vi "Dhoot Front Measurement Block.vi"(0 "Image in":T4, 1 "Coord Centre X":dbl, 2 "Measurement ROI":T10={"Left"=40.0, "Top"=75.0, "Right"=80.0, "Bottom"=3.0, "Angle"=0.0}, 3 "Coord Centre Y":dbl, 4 "Angle":dbl, 5 "ROI Enable":bool, 6 "Measu Ref Step Size":u32=1, 7 "error in (no error)":errorcluster, 8 "Measurement ROI Scan Direction":u16(ring) items=["Left To Right", "Right To Left", "Top To Bottom", "Bottom To Top"], 9 "Measurement Reference ROI":T10={"Left"=0.0, "Top"=0.0, "Right"=0.0, "Bottom"=280.0, "Angle"=0.0}, 10 "Measu ROI Process":T7(ring)=enum."Get First + Last Edge", 11 "Measu Ref Process":T7(ring), 12 "Measu ROI Step Size":u32=1, 13 "Measu Ref Edge Options":T5={"Edge Polarity"=0, "Kernel Size"=5, "Width"=5, "Minimum Edge Strength"=40.0, "Interpolation Type"=enum."Zero Order", "Data Processing Method"=enum."Average"} {"Edge Polarity" items=["All Edges", "Rising Edges", "Falling Edges"]; "Minimum Edge Strength" format="%.2f"; "Width" step=2; "Kernel Size" step=2}, 14 "Measu Edge Options":T5={"Edge Polarity"=0, "Kernel Size"=5, "Width"=5, "Minimum Edge Strength"=40.0, "Interpolation Type"=enum."Zero Order", "Data Processing Method"=enum."Average"} {"Edge Polarity" items=["All Edges", "Rising Edges", "Falling Edges"]; "Minimum Edge Strength" format="%.2f"; "Width" step=2; "Kernel Size" step=2}, 15 "Measu Ref Scan Direction":u16(ring)=2 items=["Left To Right", "Right To Left", "Top To Bottom", "Bottom To Top"], 16 "Calibration Image":T4) -> (18 "Overlay Arrows Lines":T1, 20 "Image out":T4, 21 "Measurement":sgl, 22 "Measu Ref Edge Point":cluster{"X":sgl, "Y":sgl}, 23 "First Edges":T9[](array[typedef]) {"Distance (Real-World)" format="%.2f"; "Location (Real-World)"."Y" format="%.2g"; "Location (Real-World)"."X" format="%.2f"; "Noise" format="%.2f"; "Location (Pixel)"."Y" format="%.2g"; "Location (Pixel)"."X" format="%.2f"; "Strength" format="%.2f"; "Distance (Pixel)" format="%.2f"}, 24 "Last Edges":T9[](array[typedef]) {"Distance (Real-World)" format="%.2f"; "Location (Real-World)"."Y" format="%.2g"; "Location (Real-World)"."X" format="%.2f"; "Noise" format="%.2f"; "Location (Pixel)"."Y" format="%.2g"; "Location (Pixel)"."X" format="%.2f"; "Strength" format="%.2f"; "Distance (Pixel)" format="%.2f"}, 25 "Search Lines":T8[](array[typedef]) {"Edge Info"."Distance (Real-World)" format="%.2f"; "Edge Info"."Location (Real-World)"."Y" format="%.2g"; "Edge Info"."Location (Real-World)"."X" format="%.2f"; "Edge Info"."Noise" format="%.2f"; "Edge Info"."Location (Pixel)"."Y" format="%.2g"; "Edge Info"."Location (Pixel)"."X" format="%.2f"; "Edge Info"."Strength" format="%.2f"; "Edge Info"."Distance (Pixel)" format="%.2f"}, 27 "error IO":errorcluster)   [LabVIEW 2019, in "Algorithm.lvclass"]
uses:
  FrameworkOverrides/Algorithm.lvclass
  <vilib>/vision/NI_Vision_Development_Module.lvlib
  <vilib>/vision/Image Controls.llb/IMAQ Image.ctl
  <vilib>/vision/Measure.llb/Edge New.ctl
  <vilib>/vision/Measure.llb/Search Line.ctl
  <vilib>/vision/Measure.llb/Edge Polarity.ctl
  <vilib>/vision/Measure.llb/Edge Options.ctl
panel:
  out "Second Overlay Line":T2
  out "First Overlay Line":T3
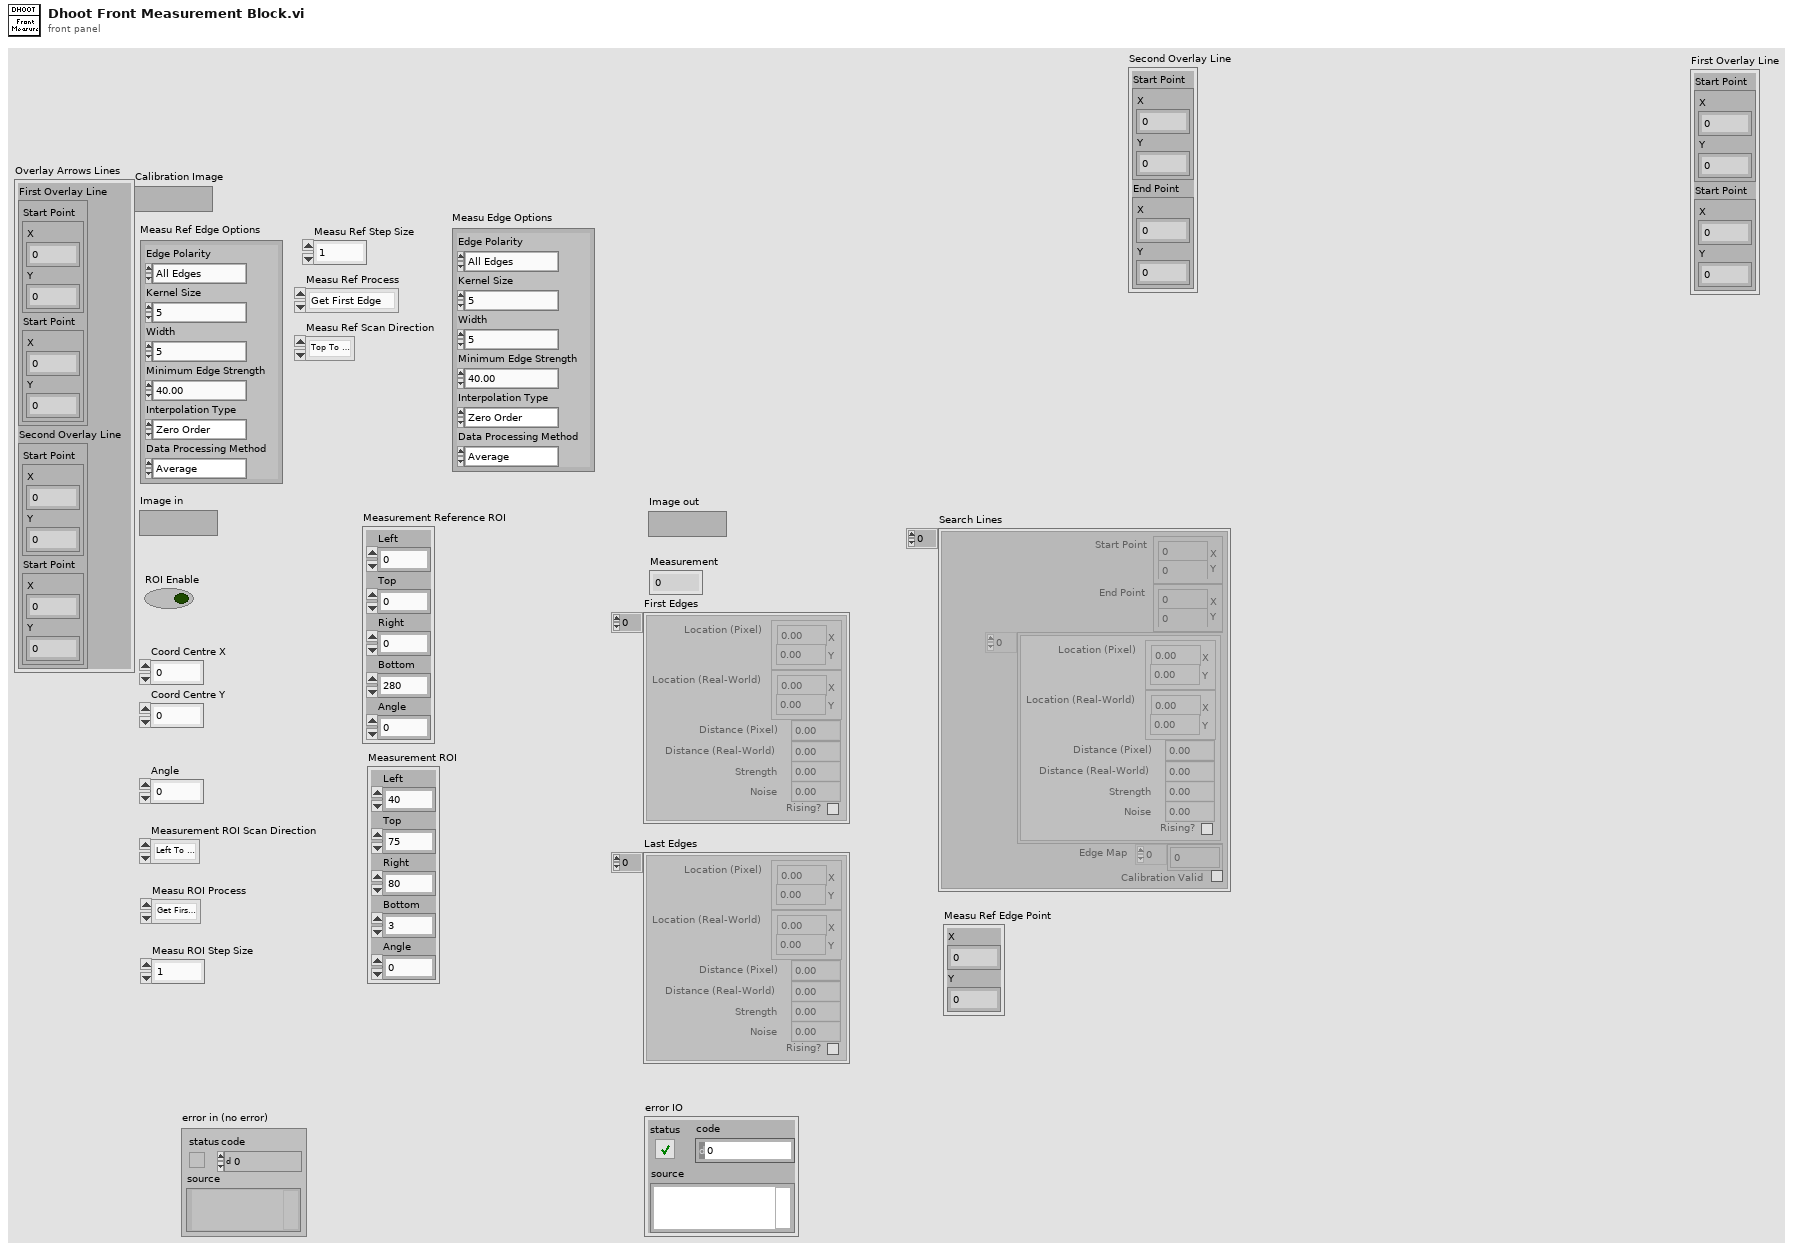
[diagram p1: front panel]
types:
  T1 = cluster{"First Overlay Line ":cluster{"Start Point":cluster{"X":sgl, "Y":sgl}, "Start Point":cluster{"X":sgl, "Y":sgl}}, "Second Overlay Line ":cluster{"Start Point":cluster{"X":sgl, "Y":sgl}, "Start Point":cluster{"X":sgl, "Y":sgl}}}
  T2 = cluster{"Start Point":cluster{"X":sgl, "Y":sgl}, "End Point":cluster{"X":sgl, "Y":sgl}}
  T3 = cluster{"Start Point":cluster{"X":sgl, "Y":sgl}, "Start Point":cluster{"X":sgl, "Y":sgl}}
  T4 = typedef "IMAQ Image.ctl" = refnum<image>
  T5 = typedef "Edge Options.ctl" = cluster{"Edge Polarity":T6, "Kernel Size":u32, "Width":u32, "Minimum Edge Strength":sgl, "Interpolation Type":enum32{"Zero Order", "Bilinear", "Quadratic", "Cubic", "Bilinear Fixed"}, "Data Processing Method":enum32{"Average", "Median"}}
  T6 = typedef "Edge Polarity.ctl" = u32
  T7 = enum16{"Get First Edge", "Get First + Last Edge", "Get All Edges", "Get Best Edge"}
  T8 = typedef "Search Line.ctl" = cluster{"Start Point":cluster{"X":sgl, "Y":sgl}, "End Point":cluster{"X":sgl, "Y":sgl}, "Edge Info":T9[], "Edge Map":dbl[], "Calibration Valid":bool}
  T9 = typedef "Edge New.ctl" = cluster{"Location (Pixel)":cluster{"X":sgl, "Y":sgl}, "Location (Real-World)":cluster{"X":sgl, "Y":sgl}, "Distance (Pixel)":dbl, "Distance (Real-World)":dbl, "Strength":dbl, "Noise":dbl, "Rising?":bool}
  T10 = cluster{"Left":dbl, "Top":dbl, "Right":dbl, "Bottom":dbl, "Angle":dbl}
  T11 = typedef "ROI Descriptor" = cluster{"Global Rectangle":i32[], "Contours":cluster{"ID":enum32{"External", "Internal"}, "Type":u32, "Coordinates":i32[]}[]}
  T12 = cluster{"Start Point":cluster{"X":sgl, "Y":sgl}, "Location (Pixel)":cluster{"X":sgl, "Y":sgl}}
  T13 = cluster{"Location (Pixel)":cluster{"X":sgl, "Y":sgl}, "End Point":cluster{"X":sgl, "Y":sgl}}
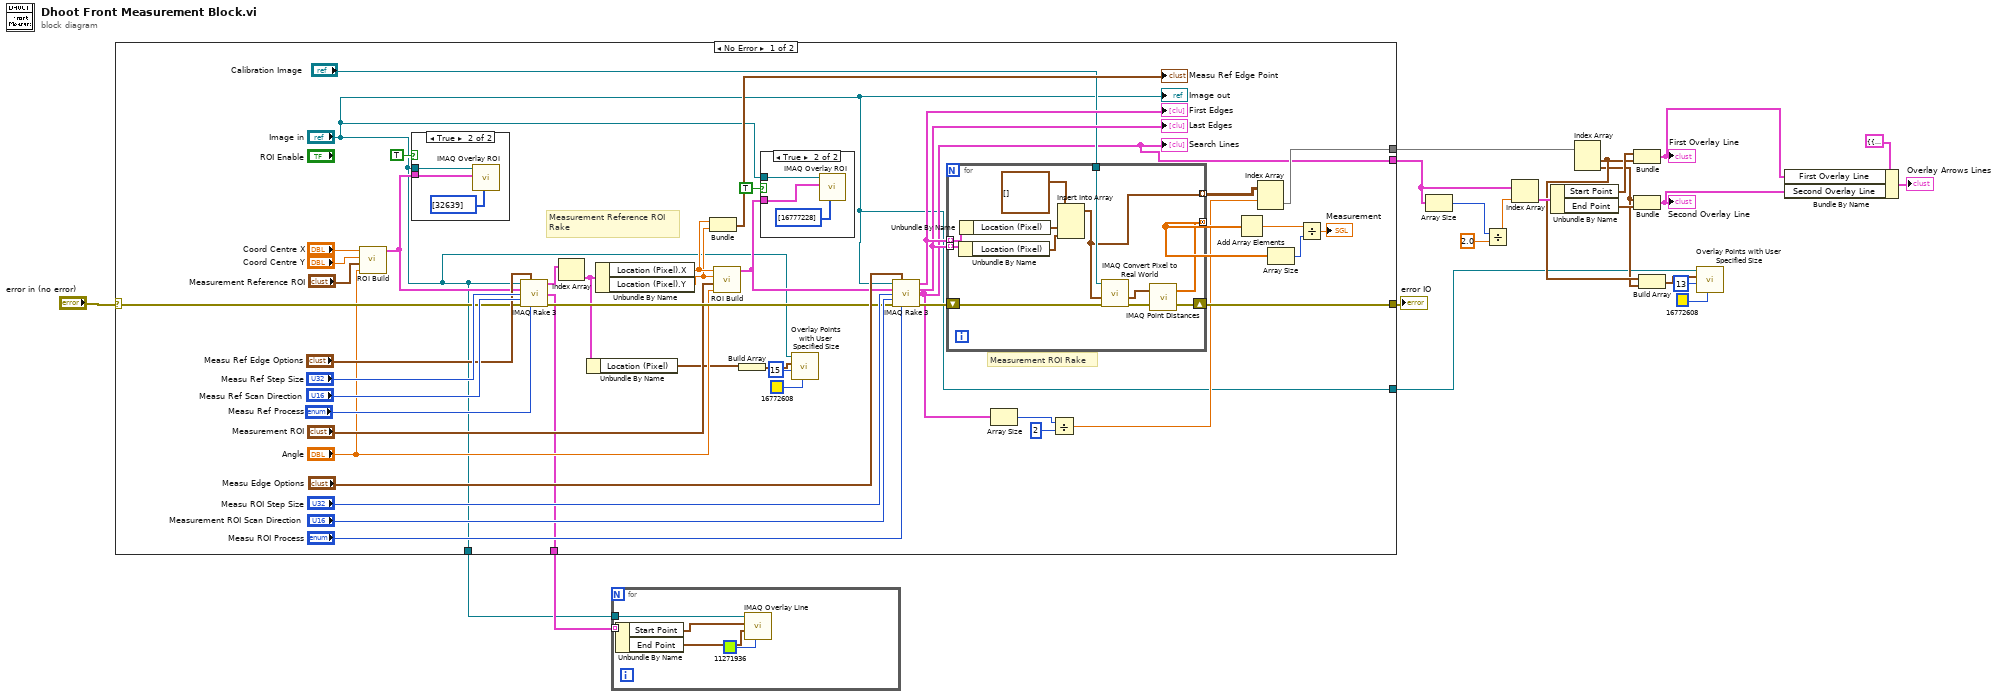
[diagram p0: block diagram]
diagram:
  n1 = case shown="No Error" "error in (no error)" {
    selector: "error in (no error)" -> [w47 w86]
    tunnel: [w38 w86] -> w21
    tunnel: [w33 _] -> w11
    tunnel: [w32 _] -> w10
    tunnel: ["Image in" _] -> w4
    tunnel: [w29 _] -> w2
    tunnel: ["Image in" _] -> w1
    frame No Error {
      # "Measurement ROI Rake"
      # "Measurement Reference ROI\nRake"
      n2 = call "ROI Build.vi"("Angle"="Angle", "input cluster"="Measurement Reference ROI", "Centre Y"="Coord Centre Y", "Centre X"="Coord Centre X") -> ("ROI Descriptor"=w63:T11)  [unwired: 7 in]
      n3 = case shown="True" TRUE {
        tunnel: w63 -> [_ w73]
        tunnel: "Image in" -> [_ w72]
        frame False {
        }
        frame True {
          n4 = call "IMAQ Overlay ROI"("Colors (Green)"=u32[] [32639], "ROI Descriptor"=w73, "Image"=w72) -> ()  [unwired: 7 in, 2 out]
        }
      }
      n5 = call "IMAQ Rake 3"("Image"="Image in", "Edge Options"="Measu Ref Edge Options", "ROI Descriptor"=w63, "Step Size"="Measu Ref Step Size", "Scan Direction"="Measu Ref Scan Direction", "error in (no error)"=w47, "Process"="Measu Ref Process") -> ("First Edges"=w62:T9[], "Search Lines"=w29:T8[], "error out"=w53:errorcluster)  [unwired: 5 in, 1 out]
      n6 = Index Array(array=w62) -> (element=w28:T9)  [unwired: 1 in]
      n7 = Unbundle By Name(w28) -> ("Location (Pixel)"=w27:cluster{"X":sgl, "Y":sgl})
      n8 = Unbundle By Name(w28) -> ("Location (Pixel).X"=w43:sgl, "Location (Pixel).Y"=w42:sgl)
      n9 = Bundle("X"=w43, "Y"=w42) -> (→"Measu Ref Edge Point":cluster{"X":sgl, "Y":sgl})  [unwired: 1 in]
      n10 = call "ROI Build.vi"("Angle"="Angle", "input cluster"="Measurement ROI", "Centre Y"=w42, "Centre X"=w43) -> ("ROI Descriptor"=w50:T11)  [unwired: 7 in]
      n11 = Build Array(w27) -> (w26:cluster{"X":sgl, "Y":sgl}[])
      n12 = case shown="True" TRUE {
        tunnel: w50 -> [_ w70]
        tunnel: "Image in" -> [_ w69]
        frame False {
        }
        frame True {
          n13 = call "IMAQ Overlay ROI"("Colors (Green)"=u32[] [16777228], "ROI Descriptor"=w70, "Image"=w69) -> ()  [unwired: 7 in, 2 out]
        }
      }
      n14 = call "Overlay Points with User Specified Size.vi"("Color"=u32 16772608, "Point Diameter (5)"=u32 15, "Points"=w26, "Image In"="Image in") -> ()  [unwired: 6 in, 2 out]
      n15 = call "IMAQ Rake 3"("Image"="Image in", "Edge Options"="Measu Edge Options", "ROI Descriptor"=w50, "Step Size"="Measu ROI Step Size", "Scan Direction"="Measurement ROI Scan Direction", "error in (no error)"=w53, "Process"="Measu ROI Process") -> ("First Edges"=w52:T9[], "Last Edges"=w51:T9[], "Search Lines"=w32:T8[], "error out"=w40:errorcluster)  [unwired: 5 in]
      "First Edges" <- w52
      "Last Edges" <- w51
      "Search Lines" <- w32
      n16 = for {
        tunnel: w52 -> [w85] mode=indexing
        tunnel: w51 -> [w84] mode=indexing
        tunnel: [w82] -> w57 mode=concatenating
        shift-right: [w77] -> w38
        shift-left: w40 -> [w79]
        tunnel: "Calibration Image" -> [w75]
        tunnel: [w74] -> w37 mode=indexing
        n17 = Unbundle By Name(w84) -> ("Location (Pixel)"=w80:cluster{"X":sgl, "Y":sgl})
        n18 = Unbundle By Name(w85) -> ("Location (Pixel)"=w81:cluster{"X":sgl, "Y":sgl})
        n19 = Insert Into Array(array=cluster{"X":sgl, "Y":sgl}[] [], new element #1=w81, new element #2=w80) -> (w74:cluster{"X":sgl, "Y":sgl}[])  [unwired: 1 in]
        n20 = call "IMAQ Convert Pixel to Real World"("error in (no error)"=w79, "Array of Pixel Coordinates"=w74, "Calibrated Image"=w75) -> ("error out"=w78:errorcluster, "Array of Real World Coordinates"=w76:cluster{"X":sgl, "Y":sgl}[])  [unwired: 3 in, 4 out]
        n21 = call "IMAQ Point Distances"("Points"=w76, "error in (no error)"=w78) -> ("Distances"=w82:sgl[], "error out"=w77:errorcluster)  [unwired: 3 in]
      }
      n22 = Array Size(array=w32) -> (size(s)=w36:i32)
      n23 = Divide(x=w36, y=2) -> (x/y=w34:dbl)
      n24 = Add Array Elements(numeric array=w57) -> (sum=w56:sgl)
      n25 = Index Array(array=w37, index (row)=w34) -> (element=w33:cluster{"X":sgl, "Y":sgl}[])  [unwired: 1 in]
      n26 = Array Size(array=w57) -> (size(s)=w55:i32)
      n27 = Divide(x=w56, y=w55) -> (x/y=→"Measurement":sgl)
      "Image out" <- "Image in"
    }
    frame Error {
    }
  }
  "error IO" <- w21
  n28 = for {
    tunnel: w2 -> [w91] mode=indexing
    tunnel: w1 -> [w88]
    n29 = Unbundle By Name(w91) -> ("Start Point"=w90:cluster{"X":sgl, "Y":sgl}, "End Point"=w89:cluster{"X":sgl, "Y":sgl})
    n30 = call "IMAQ Overlay Line"("Color"=u32 11271936, "End Point"=w89, "Start Point"=w90, "Image"=w88) -> ()  [unwired: 6 in, 2 out]
  }
  n31 = Array Size(array=w10) -> (size(s)=w13:i32)
  n32 = Divide(x=w13, y=2.0) -> (x/y=w12:dbl)
  n33 = Index Array(array=w10, index=w12) -> (element=w20:T8)
  n34 = Unbundle By Name(w20) -> ("Start Point"=w19:cluster{"X":sgl, "Y":sgl}, "End Point"=w18:cluster{"X":sgl, "Y":sgl})
  n35 = Index Array(array=w11) -> (element #1=w8:cluster{"X":sgl, "Y":sgl}, element #2=w7:cluster{"X":sgl, "Y":sgl})  [unwired: 2 in]
  n36 = Bundle("Start Point"=w19, "Location (Pixel)"=w8) -> (w16:T12)  [unwired: 1 in]
  "First Overlay Line" <- w16
  n37 = Bundle("Location (Pixel)"=w7, "End Point"=w18) -> (w15:T13)  [unwired: 1 in]
  "Second Overlay Line" <- w15
  n38 = Build Array(w8, w7) -> (w6:cluster{"X":sgl, "Y":sgl}[])
  n39 = call "Overlay Points with User Specified Size.vi"("Color"=u32 16772608, "Point Diameter (5)"=u32 13, "Points"=w6, "Image In"=w4) -> ()  [unwired: 6 in, 2 out]
  n40 = Bundle By Name(cluster=T1 {"First Overlay Line "={"Start Point"={"X"=0.0, "Y"=0.0}, "Start Point"={"X"=0.0, "Y"=0.0}}, "Second Overlay Line "={"Start Point"={"X"=0.0, "Y"=0.0}, "Start Point"={"X"=0.0, "Y"=0.0}}}, "First Overlay Line"=w16, "Second Overlay Line"=w15) -> (→"Overlay Arrows Lines":T1)
